vi "Message encoder.vi"(8 "error in (no error)":errorcluster, 10 "Data":variant, 11 "Kasli Writer in":refnum<class "Kasli Writer.lvclass">) -> (0 "error out":errorcluster, 2 "Message encoded":string, 3 "Kasli Writer out":refnum<class "Kasli Writer.lvclass">)   [LabVIEW 2020, in "Kasli Listener and Writer.lvlib" / "Kasli Writer.lvclass"]
uses:
  Kasli Writer.lvclass
  Ancestor/Ancestor/Ancestor.lvclass/Ancestor.ctl
  Support VIs/Generate Error.vi
  FGV/Error Memory/Get Error Description.vi
  Support VIs/Get PC name.vi
  Ancestor/Ancestor/Read ID.vi
  Support VIs/Get Class Name.vi
  <vilib>/Utility/error.llb/Clear Errors.vi
  FGV/Error Memory/Error Memory Core.vi
  <vilib>/AdvancedString/Delimited String to 1D String Array.vi
  Support VIs/Circus Root Path.vi
  FGV/Error Memory/Error Crt Lvl checker.vi
  FGV/Error Memory/Error Memory Core.vi/40c8088d-b597-4017-91af-faa98e00292e.vi
  FGV/Error Memory/Error Memory Core.vi/d4a3ab98-063c-4e44-b43d-fbdcfe6c2be2.vi
  Support VIs/Global Memory.vi
  <vilib>/Utility/LVClass/Get LV Class Name.vi
  Support VIs/Is in Packed Library.vi
  Support VIs/TALOS Root path.vi
  Support VIs/Read CSV worksheet.vi
  Support VIs/Global Constants.vi
  <vilib>/Utility/error.llb/General Error Handler.vi
  Support VIs/Error Log.vi
  Ancestor/Ancestor/Ancestor.lvclass
  <vilib>/Comparison/Equal/Equal Functor/Equal Functor.lvclass
  TALOS.lvlib
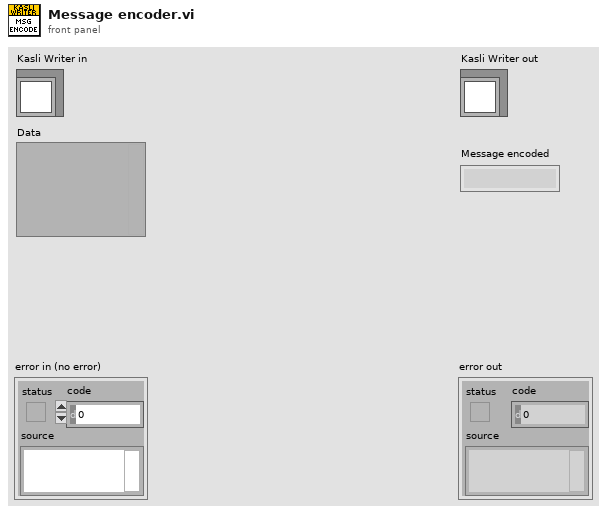
[diagram p1: front panel]
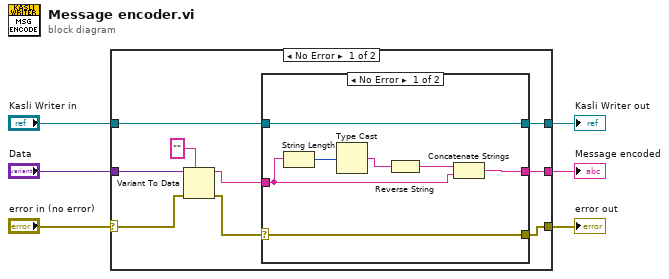
[diagram p0: block diagram]
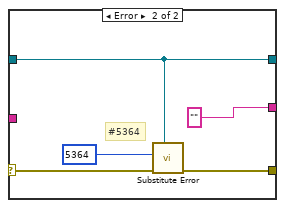
[diagram p2: hidden frame]
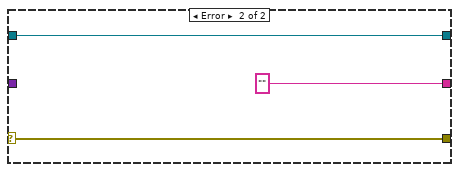
[diagram p3: hidden frame]
diagram:
  n1 = case shown="No Error" "error in (no error)" {
    selector: "error in (no error)" -> [w13 w28]
    tunnel: "Data" -> [w15 _]
    tunnel: [w7 ""] -> w5
    tunnel: [w8 w28] -> w3
    tunnel: "Kasli Writer in" -> [w12 w30]
    tunnel: [w11 w30] -> w1
    frame No Error {
      n2 = Variant To Data(error in=w13, type="", Variant=w15) -> (data=w10:string, error out=w9:errorcluster)
      n3 = case shown="No Error" w9 {
        selector: w9 -> [w18 w25]
        tunnel: [w22 w26] -> w11
        tunnel: w12 -> [w22 w26]
        tunnel: w10 -> [w20 _]
        tunnel: [w19 ""] -> w7
        tunnel: [w18 w24] -> w8
        frame No Error {
          n4 = String Length(string=w20) -> (length=w17:i32)
          n5 = Type Cast(x=w17) -> (*(type *) &x=w21:string)  [unwired: 1 in]
          n6 = Reverse String(1:w21) -> (0:w16:string)
          n7 = Concatenate Strings(w16, w20) -> (w19:string)
        }
        frame Error {
          # "#5364"
          n8 = call "Substitute Error.vi"("LabVIEW Object"=w26, "error in (no error)"=w25, "Error Code"=5364) -> ("error out"=w24:errorcluster)  [unwired: 8 in]
        }
      }
    }
    frame Error {
    }
  }
  "error out" <- w3
  "Kasli Writer out" <- w1
  "Message encoded" <- w5
